vi "LiveAcquireOlder.vi"() -> ()   [LabVIEW 2015]
uses:
  LiveImage_Global.vi
  NIDAQControls/NIDAQGlobals.vi
panel:
  out "error out 3":errorcluster
  out "Acquire Time":dbl
  out "Wait Time":dbl
  in  "error out":errorcluster
  out "ypixels":i32
  out "xpixels":i32
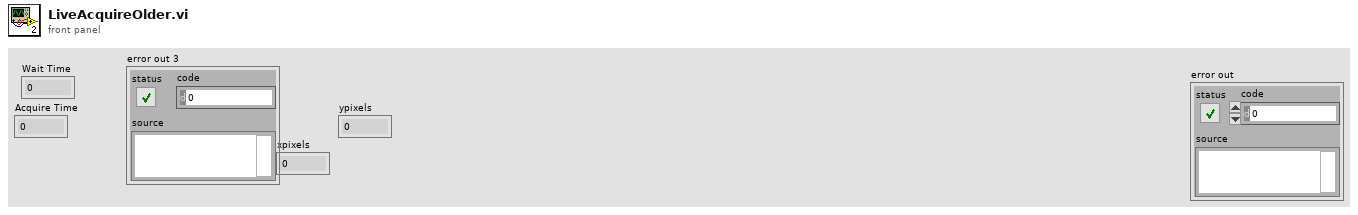
[diagram p1: front panel]
types:
  T1 = typedef "Rendezvous RefNum" = refnum<k1>
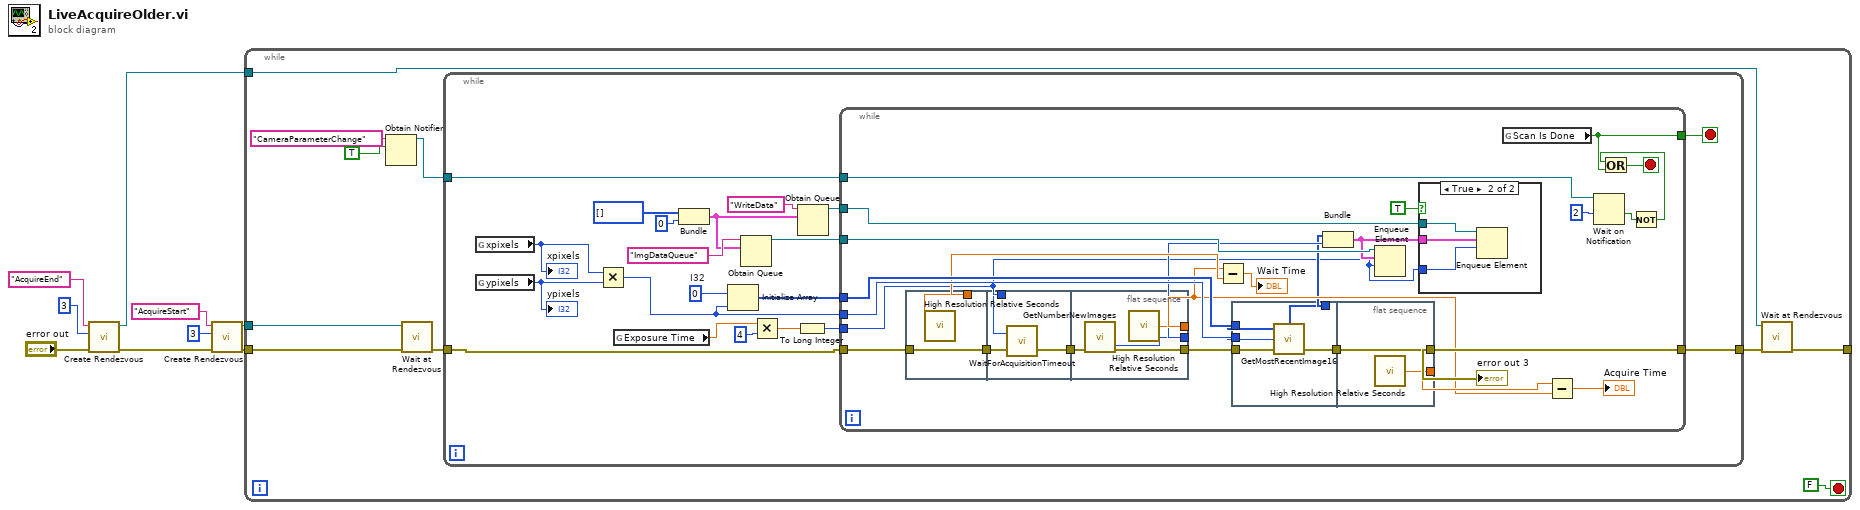
[diagram p0: block diagram]
diagram:
  n1 = call <vilib>:"Create Rendezvous.vi"("error in (no error)"="error out", "size (2)"=3, "name (unnamed)"="AcquireEnd") -> ("error out"=w2:errorcluster, "rendezvous"=w8:T1)  [unwired: 2 in, 1 out]
  n2 = call <vilib>:"Create Rendezvous.vi"("error in (no error)"=w2, "size (2)"=3, "name (unnamed)"="AcquireStart") -> ("error out"=w1:errorcluster, "rendezvous"=w4:T1)  [unwired: 2 in, 1 out]
  n3 = while {
    tunnel: [w15] -> _
    tunnel: w1 -> [w19]
    tunnel: w8 -> [w13]
    tunnel: w4 -> [w16]
    stop <- FALSE stop-if-true
    n4 = Obtain Notifier(name (unnamed)="CameraParameterChange", notification data type=TRUE) -> (notifier out=w10:refnum<notifier>)  [unwired: 2 in, 2 out]
    n5 = call <vilib>:"Wait at Rendezvous.vi"("error in (no error)"=w19, "rendezvous"=w16) -> ("error out"=w14:errorcluster)  [unwired: 3 in, 2 out]
    n6 = while {
      tunnel: w10 -> [w20]
      tunnel: w14 -> [w26]
      tunnel: [w39] -> w17
      stop <- w21 stop-if-true
      w38 = u16 0  # I32
      n7 = global read "LiveImage_Global.vi" "xpixels"() -> (w36:i32)
      "xpixels" <- w36
      n8 = global read "LiveImage_Global.vi" "ypixels"() -> (w37:i32)
      "ypixels" <- w37
      n9 = Multiply(x=w36, y=w37) -> (x*y=w30:i32)
      n10 = global read "LiveImage_Global.vi" "Exposure Time"() -> (w33:dbl)
      n11 = Bundle(u16[] [], 0) -> (w22:cluster{u16[], i32})  [unwired: 1 in]
      n12 = Initialize Array "Initialize Array"(w38, w30) -> (w35:u16[])
      n13 = Obtain Queue(name (unnamed)="ImgDataQueue", element data type=w22) -> (queue out=w27:refnum<queue>)  [unwired: 3 in, 2 out]
      n14 = Multiply(x=w33, y=4) -> (x*y=w32:dbl)
      n15 = To Long Integer(number=w32) -> (32bit integer=w31:i32)
      n16 = Obtain Queue(name (unnamed)="WriteData", element data type=w22) -> (queue out=w23:refnum<queue>)  [unwired: 3 in, 2 out]
      n17 = while {
        tunnel: [w65] -> w39
        tunnel: w30 -> [w60]
        tunnel: w35 -> [w59]
        tunnel: w31 -> [w46]
        tunnel: w27 -> [w53]
        tunnel: w26 -> [w50]
        tunnel: w23 -> [w48]
        tunnel: [w45] -> w21
        tunnel: w20 -> [w43]
        stop <- w44 stop-if-true
        n18 = flat-sequence {
          tunnel: w50 -> [w70]
          tunnel: [w70] -> w62
          tunnel: [w69] -> w58
          tunnel: w62 -> [w73]
          tunnel: [w72] -> w61
          tunnel: w46 -> [w71]
          tunnel: [w75] -> w64
          tunnel: w61 -> [w76]
          tunnel: [w77] -> w54
          tunnel: [w74] -> w52
          frame #0 {
            n19 = call <vilib>:"High Resolution Relative Seconds.vi"() -> ("relative seconds"=w69:dbl)
          }
          frame #1 {
            n20 = call <userlib>:"WaitForAcquisitionTimeout.vi"("error in (no error)"=w73, "iTimeOutMs"=w71) -> ("error out"=w72:errorcluster)  [unwired: 1 out]
          }
          frame #2 {
            n21 = call <userlib>:"GetNumberNewImages.vi"("error in (no error)"=w76) -> ("error out"=w75:errorcluster, "last"=w74:i32)  [unwired: 3 in, 2 out]
            n22 = call <vilib>:"High Resolution Relative Seconds.vi"() -> ("relative seconds"=w77:dbl)
          }
        }
        n23 = Subtract(x=w54, y=w58) -> (x-y=→"Wait Time":dbl)
        n24 = flat-sequence {
          tunnel: w60 -> [w82]
          tunnel: w59 -> [w81]
          tunnel: [w79] -> w51
          tunnel: [w80] -> w63
          tunnel: w64 -> [w78]
          tunnel: [w84] -> w65
          tunnel: w63 -> [w84]
          tunnel: [w83] -> w55
          frame #0 {
            n25 = call <userlib>:"GetMostRecentImage16.vi"("error in (no error)"=w78, "size"=w82, "array"=w81) -> ("error out"=w80:errorcluster, "array"=w79:u16[])  [unwired: 1 out]
          }
          frame #1 {
            n26 = call <vilib>:"High Resolution Relative Seconds.vi"() -> ("relative seconds"=w83:dbl)
          }
        }
        n27 = Bundle("array"=w51, "last"=w52) -> (w47:cluster{"array":u16[], "last":i32})  [unwired: 1 in]
        n28 = Enqueue Element(queue=w53, element=w47, timeout in ms (-1)=w46) -> ()  [unwired: 1 in, 3 out]
        n29 = case shown="True" TRUE {
          tunnel: w48 -> [_ w68]
          tunnel: w47 -> [_ w67]
          tunnel: w46 -> [_ w66]
          frame False {
          }
          frame True {
            n30 = Enqueue Element(queue=w68, element=w67, timeout in ms (-1)=w66) -> ()  [unwired: 1 in, 3 out]
          }
        }
        n31 = global read "NIDAQGlobals.vi" "Scan Is Done"() -> (w45:bool)
        n32 = Subtract(x=w55, y=w54) -> (x-y=→"Acquire Time":dbl)
        n33 = Wait on Notification(notifier=w43, timeout in ms (-1)=2) -> (timed out?=w41:bool)  [unwired: 2 in, 3 out]
        n34 = Not(x=w41) -> (.not. x?=w40:bool)
        n35 = Or(x=w40, y=w45) -> (x .or. y?=w44:bool)
        "error out 3" <- w65
      }
    }
    n36 = call <vilib>:"Wait at Rendezvous.vi"("error in (no error)"=w17, "rendezvous"=w13) -> ("error out"=w15:errorcluster)  [unwired: 3 in, 2 out]
  }
